vi "inittrv2.vi"(8 "OptsVer":string="default", 9 "Write/Read":u16(ring) items=["Write", "Read"], 10 "CtlRefs":refnum<vi>[](array[refnum]), 11 "Main VI":refnum<vi>) -> ()   [LabVIEW 2014]
uses:
  <vilib>/Utility/config.llb/Read Key (Double).vi
  <vilib>/Utility/config.llb/Write Key (Double).vi
  <vilib>/Utility/config.llb/NI_LVConfig.lvlib
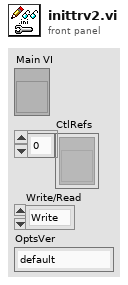
[diagram p1: front panel]
types:
  T1 = typedef "NI_LVConfig.lvlib/Config Data RefNum.ctl" = refnum<k1>
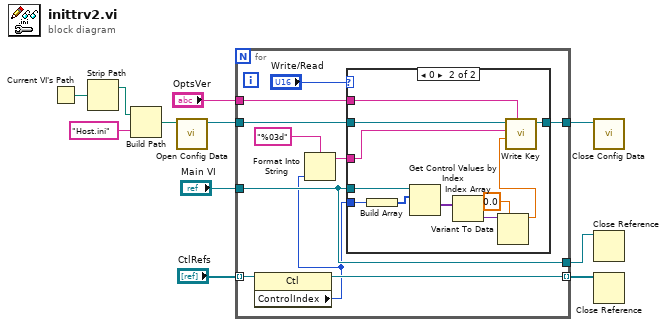
[diagram p0: block diagram]
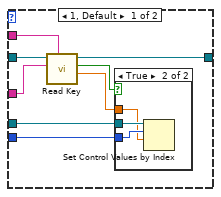
[diagram p2: hidden frame]
diagram:
  n1 = Current VI's Path() -> (path=w11:path)
  n2 = Strip Path(path=w11) -> (stripped path=w10:path)  [unwired: 1 out]
  n3 = Build Path(base path=w10, name or relative path="Host.ini") -> (appended path=w8:path)
  n4 = call <vilib>:"Open Config Data.vi"("configuration file path"=w8) -> ("refnum"=w1:T1)  [unwired: 8 in, 2 out]
  n5 = for {
    tunnel: w1 -> [w19]
    tunnel: "CtlRefs" -> [w21] mode=indexing
    tunnel: [w20] -> w3 mode=indexing
    tunnel: [w18] -> w4
    tunnel: "OptsVer" -> [w17]
    tunnel: "Main VI" -> [w16]
    tunnel: [w16] -> w2
    n6 = property class="Ctl"(reference=w21) -> (reference out=w20:refnum<vi>, "ControlIndex"=w13:i32)  [unwired: 1 in, 1 out]
    n7 = Format Into String(format string="%03d", w13) -> (resulting string=w12:string)  [unwired: 2 in, 1 out]
    n8 = case shown="0" "Write/Read" {
      tunnel: w19 -> [w29 w43]
      tunnel: [w28 w42] -> w18
      tunnel: w17 -> [w27 w41]
      tunnel: w13 -> [w24 w40]
      tunnel: w16 -> [w25 w34]
      tunnel: w12 -> [w22 w33]
      frame 1, Default {
        n9 = call-poly <vilib>:"Read Key.vi"("section"=w27, "key"=w22, "refnum"=w29) -> ("value"=w23:dbl, "found?"=w26:bool, "refnum out"=w28:T1)  [unwired: 5 in, 1 out]
        n10 = case shown="True" w26 {
          tunnel: w25 -> [_ w32]
          tunnel: w24 -> [_ w31]
          tunnel: w23 -> [_ w30]
          frame False {
          }
          frame True {
            n11 = Set Control Values by Index(0:w32, 1:w31, 2:w30) -> ()  [unwired: 1 in, 1 out]
          }
        }
      }
      frame 0 {
        n12 = Build Array(w40) -> (w39:i32[])
        n13 = Get Control Values by Index(0:w34, 1:w39) -> (10:w38:variant[])  [unwired: 1 in, 1 out]
        n14 = Index Array(array=w38) -> (element=w37:variant)  [unwired: 1 in]
        n15 = Variant To Data(type=0.0, Variant=w37) -> (data=w35:dbl)  [unwired: 1 in, 1 out]
        n16 = call-poly <vilib>:"Write Key.vi"("section"=w41, "value"=w35, "key"=w33, "refnum"=w43) -> ("refnum out"=w42:T1)  [unwired: 5 in, 2 out]
      }
    }
  }
  n17 = call <vilib>:"Close Config Data.vi"("refnum"=w4) -> ()  [unwired: 9 in, 2 out]
  n18 = Close Reference(reference=w2) -> ()  [unwired: 1 in, 1 out]
  n19 = Close Reference(reference=w3) -> ()  [unwired: 1 in, 1 out]
